vi "坐标输入子VI.vi"() -> (0 "生成的波形":waveform(dbl)(graph), 1 "最小值":dbl format="%#_3g", 2 "最大值":dbl format="%#_3g", 3 "频率":dbl)   [LabVIEW 2017]
uses:
  <vilib>/gmath/NI_Gmath.lvlib
panel:
  in  "选项卡控件":enum32{"参数设置与波形显示", "使用说明"}(tab)
  in  "输入时间t":dbl[](array[numeric]) min=0.0 step=0.0001
  in  "输入值y":dbl[](array[numeric]) min=-10.0 max=10.0
  in  "终止时间(s)":dbl min=0.0
  in  "完成":bool
  in  "插值方式":u16(ring) items=["最近", "线性", "样条插值", "cubic Hermite", "拉格朗日"]
  # "坐 标 输 入"
  # "说明：\n1、先设置“终止时间”，然后输入“输入时间（t）”和“输入值”，并且选择“插值方式”；\n2、输入时间必须以0开始，以终止时间结束，输入的时间尽量从小到大排列，且尽量均匀取间隔；\n3、当运行程序，这是“终止时间”、输入时间（t）”和“输入值”已经被程序初始化，设了一些默认的值，\n      可以在此基础上进行修改，改成符合实际需求的数值；\n4、如果采用程序初始化的值，这事波形图区并没有显示出应有的波形，这时，可以改变“输入时间（t）”、\n“输入值”和“插值方式”的值，波形图区就会显示出波形了。\n5、如果改变“终止时间”的值，则波形图区会清零，这时再重复3和4步，就可以生成新的波形了。"
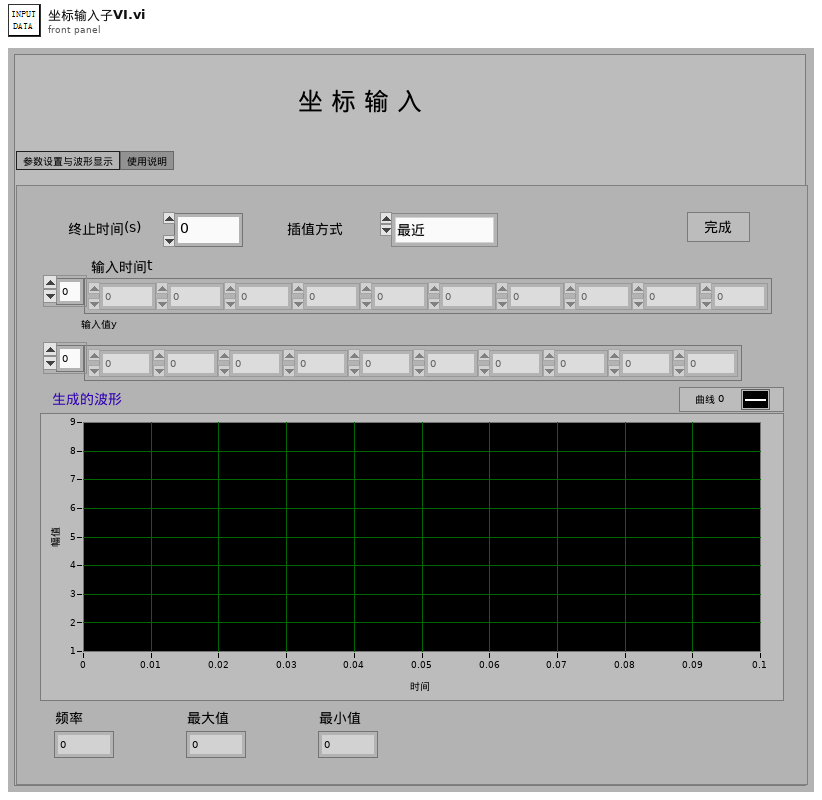
[diagram p1: front panel]
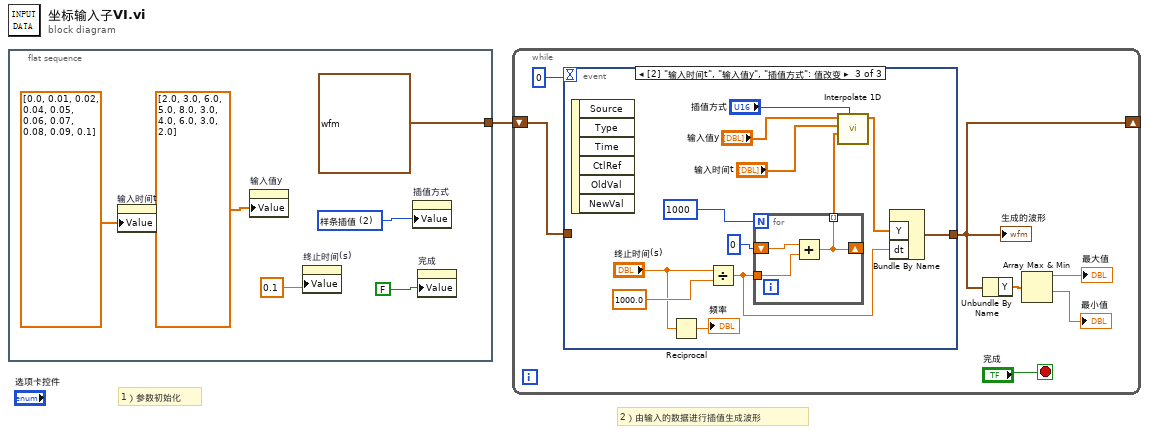
[diagram p0: block diagram]
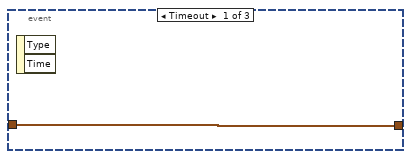
[diagram p2: hidden frame]
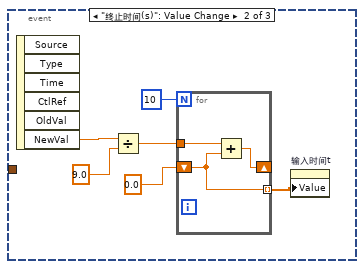
[diagram p3: hidden frame]
diagram:
  # "2）由输入的数据进行插值生成波形"
  # "1）参数初始化"
  n1 = flat-sequence {
    tunnel: [waveform(dbl) {"t0"=timestamp(0 s since 1904-01-01), "dt"=1.0, "Y"=[0.0, 0.0]} ("resampled waveform out")] -> w1
    frame #0 {
      w4 = u16 2 items=["最近", "线性", "样条插值", "cubic Hermite", "拉格朗日"] ("插值方式")
      n2 = property on="输入时间t" class="Arr (严格)"("Value"=dbl[] [0.0, 0.01, 0.02, 0.04, 0.05, 0.06, 0.07, 0.08, 0.09, 0.1] ("输入时间t")) -> ()  [unwired: 2 in, 2 out]
      n3 = property on="输入值y" class="Arr (严格)"("Value"=dbl[] [2.0, 3.0, 6.0, 5.0, 8.0, 3.0, 4.0, 6.0, 3.0, 2.0] ("输入值y")) -> ()  [unwired: 2 in, 2 out]
      n4 = property on="终止时间(s)" class="DigNum (严格)"("Value"=0.1 ("终止时间(s)")) -> ()  [unwired: 2 in, 2 out]
      n5 = property on="插值方式" class="Ring (严格)"("Value"=w4) -> ()  [unwired: 2 in, 2 out]
      n6 = property on="完成" class="Bool (严格)"("Value"=FALSE ("确定按钮")) -> ()  [unwired: 2 in, 2 out]
    }
  }
  n7 = while {
    shift-right: [w8] -> _
    shift-left: w1 -> [w12]
    stop <- "完成" stop-if-true
    n8 = event shown="[2] \"输入时间t\", \"输入值y\", \"插值方式\": 值改变" {
      selector: _ -> [_ _ _]
      dyn-events: _ -> [_ _ _]
      timeout: 0 -> [_ _ _]
      tunnel: [w15 _ w28] -> w8
      tunnel: w12 -> [w15 _ _]
      event Timeout {
        n9 = event-data() -> ()  [unwired: 1 in, 2 out]
      }
      event "终止时间(s)": Value Change {
        n10 = event-data() -> ("NewVal"=w21:dbl)  [unwired: 1 in, 5 out]
        n11 = Divide(x=w21, y=9.0) -> (x/y=w19:dbl)
        n12 = for {
          N: 10 -> [_]
          shift-right: [w23] -> _
          shift-left: 0.0 -> [w22]
          tunnel: w19 -> [w24]
          tunnel: [w22] -> w17 mode=indexing
          n13 = Add(x=w24, y=w22) -> (x+y=w23:dbl)
        }
        n14 = property on="输入时间t" class="Arr (严格)"("Value"=w17) -> ()  [unwired: 2 in, 2 out]
      }
      event "输入时间t", "输入值y", "插值方式": Value Change {
        n15 = event-data() -> ()  [unwired: 1 in, 6 out]
        n16 = Reciprocal(x="终止时间(s)") -> (1/x=→"频率":dbl)
        n17 = Divide(x="终止时间(s)", y=1000.0) -> (x/y=w36:dbl)
        n18 = for {
          N: 1000 -> [_]
          shift-right: [w37] -> _
          shift-left: 0 -> [w38]
          tunnel: w36 -> [w39]
          tunnel: [w37] -> w25 mode=indexing
          n19 = Add(x=w38, y=w39) -> (x+y=w37:dbl)
        }
        n20 = call <vilib>:"Interpolate 1D.vi"("method"="插值方式", "xi"=w25, "X"="输入时间t", "Y"="输入值y") -> ("yi"=w35:dbl[])  [unwired: 5 in, 2 out]
        n21 = Bundle By Name("Y"=w35, "dt"=w36) -> (w28:waveform(dbl))  [unwired: 1 in]
      }
    }
    "生成的波形" <- w8
    n22 = Unbundle By Name(w8) -> ("Y"=w9:dbl[])
    n23 = Array Max & Min(array=w9) -> (max value=→"最大值":dbl, min value=→"最小值":dbl)  [unwired: 2 out]
  }
